vi "TIO RPC Send REQuest.vi"(8 "error in (no error)":errorcluster, 9 "Payload":string, 10 "Topic":string, 11 "TS Connection":T1={"Type"=enum."TCP", "Serial"="serial:///dev/cu.usbserial-00000", "TCP"=refnum, "Timeout"=500}) -> (0 "error out":errorcluster, 2 "Request ID":u16=60741 format="%04x", 3 "TS Connection":T1={"Type"=enum."TCP", "Serial"="serial:///dev/cu.usbserial-00000", "TCP"=refnum, "Timeout"=500})   [LabVIEW 2017]
uses:
  <instrlib>/tio-labview/TIO Library/Socket/Helpers/TIO SLIP Serial Write.vi
  <instrlib>/tio-labview/TIO Library/Socket/Helpers/TIO Form Packet.vi
  <instrlib>/tio-labview/TIO Library/Socket/Helpers/TIO SLIP Encode.vi
  <instrlib>/tio-labview/TIO Library/Socket/Helpers/TIO Serial Checksum CRC32.vi
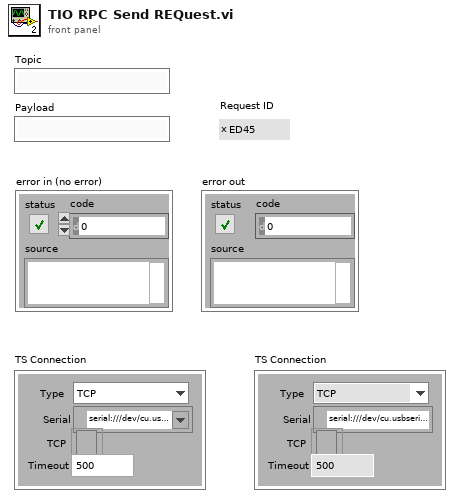
[diagram p1: front panel]
types:
  T1 = cluster{"Type":enum16{"TCP", "Serial"}, "Serial":refnum<visa-resource-name>, "TCP":refnum<k5>, "Timeout":u32}
  T2 = enum8{"Invalid", "Log", "RPC Request", "RPC Reply", "RPC Error", "Stream Description", "User"}
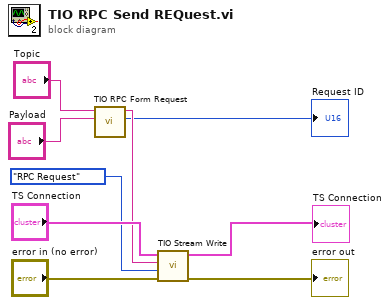
[diagram p0: block diagram]
diagram:
  n1 = call <instrlib>:"TIO RPC Form Request.vi"("Payload"="Payload", "Topic"="Topic") -> ("Request ID"=→"Request ID":u16, "String out"=w3:string)  [unwired: 8 in]
  n2 = call <instrlib>:"TIO Stream Write.vi"("error in (no error)"="error in (no error)", "Type"=T2."RPC Request", "Payload"=w3, "TS Connection"="TS Connection") -> ("error out"=→"error out":errorcluster, "TS Connection"=→"TS Connection":T1)  [unwired: 5 in]
